vi "Set Loop Period.vi"(8 "error in (no error)":errorcluster, 10 "Loop Period in ms (10)":u32=10, 11 "PID Loop in":refnum<class "PID Loop.lvclass">) -> (0 "error out":errorcluster, 3 "PID Loop out":refnum<class "PID Loop.lvclass">)   [LabVIEW 2024, in "PID Loop.lvlib" / "PID Loop.lvclass"]
uses:
  PID Loop.lvclass
  PID Loop.lvclass/PID Loop.ctl
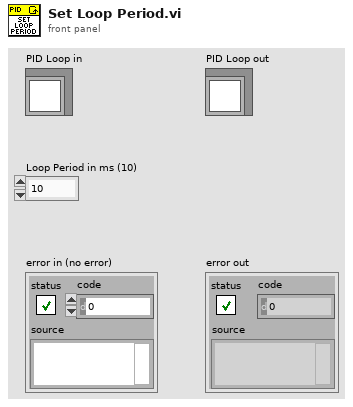
[diagram p1: front panel]
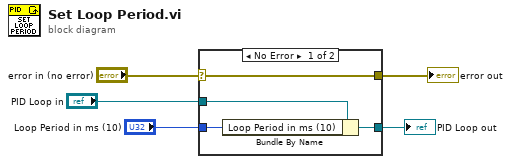
[diagram p0: block diagram]
diagram:
  n1 = case shown="No Error" "error in (no error)" {
    selector: "error in (no error)" -> [w9 w11]
    tunnel: [w9 w11] -> w4
    tunnel: [w7 w10] -> w2
    tunnel: "PID Loop in" -> [w8 w10]
    tunnel: "Loop Period in ms (10)" -> [w6 _]
    frame No Error {
      n2 = Bundle By Name(cluster=w8, "Loop Period in ms (10)"=w6) -> (w7:refnum<class "PID Loop.lvclass">)
    }
    frame Error {
    }
  }
  "error out" <- w4
  "PID Loop out" <- w2
